vi "Convert Array to Image (Cam2) (SubVI).vi"(5 "Image Size":T2={"Height"=512, "Width"=512} {"Width" step=8; "Height" step=8}, 7 "Mode":enum16{"Camera", "Video"}(ring), 11 "Data In":T1) -> (0 "Compressed Image Size (%)":dbl, 3 "Image Out":T3)   [LabVIEW 2014]
uses:
  <vilib>/vision/Image Controls.llb/IMAQ Image.ctl
  Controls (HOST)/Image Size.ctl
  Controls (HOST)/Data to Disk Bundle.ctl
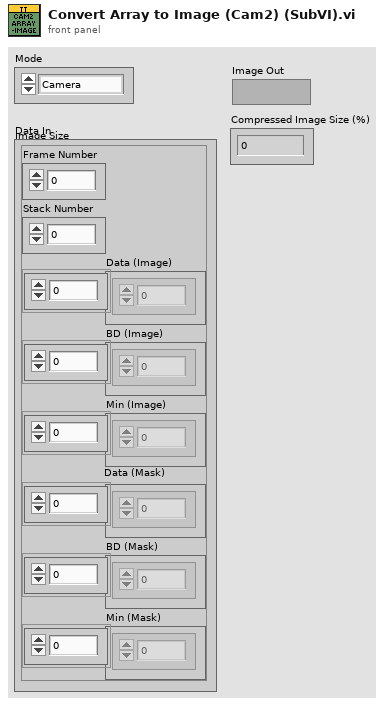
[diagram p1: front panel]
types:
  T1 = typedef "Data to Disk Bundle.ctl" = cluster{"Frame Number":u64, "Stack Number":u64, "Data (Image)":u64[], "BD (Image)":u8[], "Min (Image)":u8[], "Data (Mask)":u64[], "BD (Mask)":u8[], "Min (Mask)":u8[]}
  T2 = typedef "Image Size.ctl" = cluster{"Height":u16, "Width":u16}
  T3 = typedef "IMAQ Image.ctl" = refnum<image>
  T4 = enum16{"big-endian, network order", "native, host order", "little-endian"}
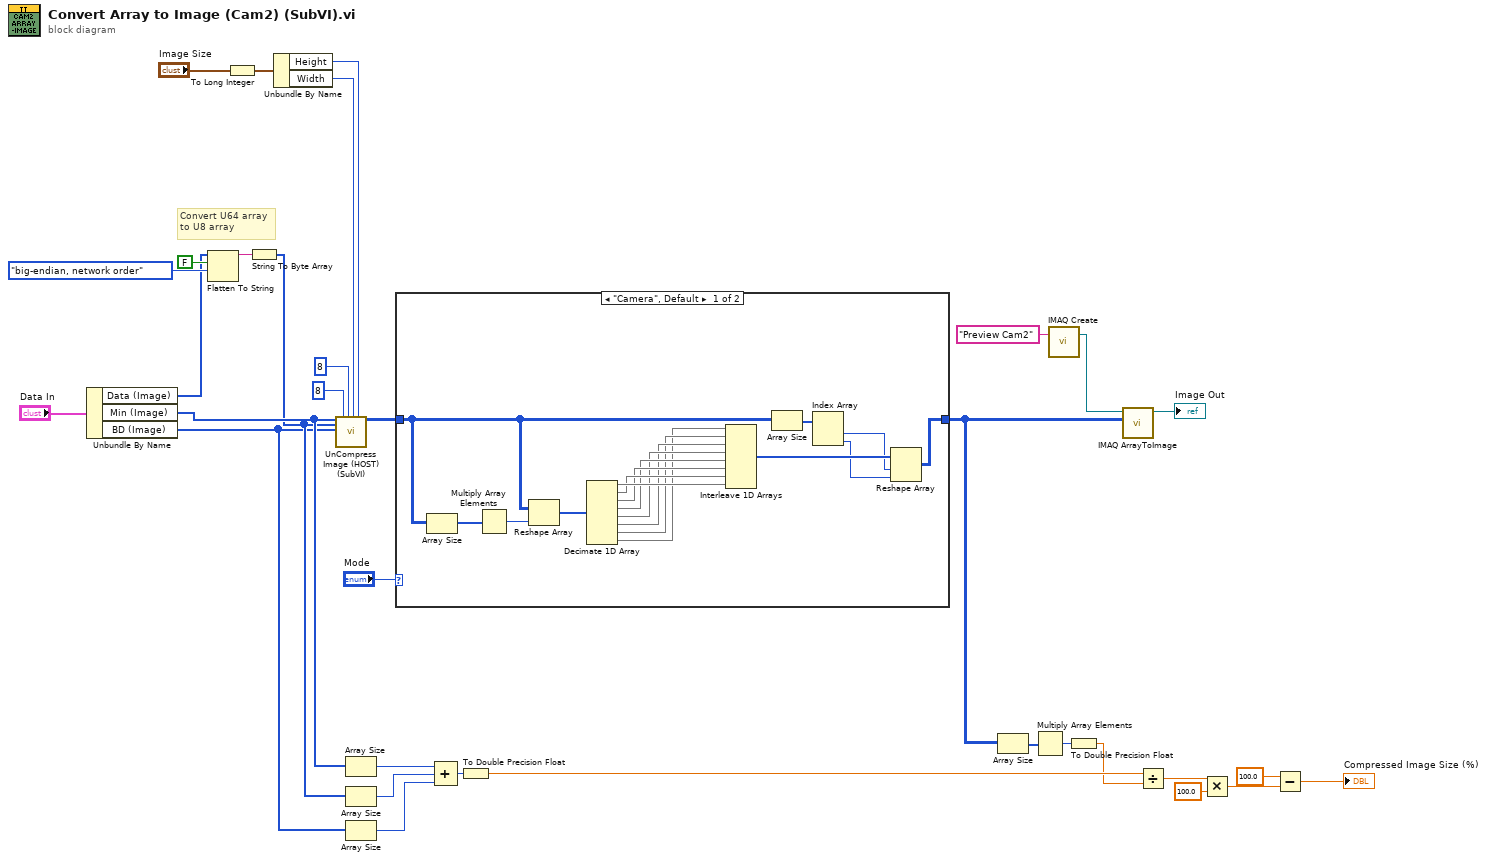
[diagram p0: block diagram]
diagram:
  # "Convert U64 array\nto U8 array"
  n1 = Unbundle By Name("Data In") -> ("Data (Image)"=w26:u64[], "Min (Image)"=w5:u8[], "BD (Image)"=w3:u8[])
  n2 = Flatten To String(anything=w26, prepend array or string size? (T)=FALSE, byte order (0:big-endian, network order)=T4."big-endian, network order") -> (data string=w28:string)  [unwired: 1 in, 2 out]
  n3 = To Long Integer(number="Image Size") -> (32bit integer=w22:cluster{"Height":i32, "Width":i32})
  n4 = String To Byte Array(string=w28) -> (unsigned byte array=w4:u8[])
  n5 = Unbundle By Name(w22) -> ("Height"=w21:i32, "Width"=w23:i32)
  n6 = call "UnCompress Image (HOST) (SubVI).vi"("Data Array"=w5, 1:w4, "Min. Array"=w3, "N Bits/Pixel"=u8 8, "Block Size"=8, "Image Width"=w23, "Image Height"=w21) -> ("Image Array Out"=w18:u8[][])  [unwired: 11 in, 1 out]
  n7 = Array Size(array=w5) -> (size(s)=w17:i32)
  n8 = Array Size(array=w4) -> (size(s)=w16:i32)
  n9 = Array Size(array=w3) -> (size(s)=w15:i32)
  n10 = case shown="\"Camera\", Default" "Mode" {
    tunnel: w18 -> [w38 w51]
    tunnel: [w34 w51] -> w6
    frame "Camera", Default {
      n11 = Array Size(array=w38) -> (size(s)=w50:i32[])
      n12 = Multiply Array Elements(1:w50) -> (0:w49:i32)
      n13 = Reshape Array(w38, w49) -> (w48:u8[])
      n14 = Decimate 1D Array(w48) -> (w47:u8[], w46:u8[], w45:u8[], w44:u8[], w43:u8[], w42:u8[], w41:u8[], w40:u8[])
      n15 = Interleave 1D Arrays(w40, w41, w42, w43, w44, w45, w46, w47) -> (w39:u8[])
      n16 = Array Size(array=w38) -> (size(s)=w37:i32[])
      n17 = Index Array(array=w37) -> (element #1=w36:i32, element #2=w35:i32)  [unwired: 2 in]
      n18 = Reshape Array(w39, w36, w35) -> (w34:u8[][])
    }
    frame "Video" {
    }
  }
  n19 = Compound Arithmetic op=ADD(w17, w16, w15) -> (w14:i32)
  n20 = To Double Precision Float(number=w14) -> (double precision float=w13:dbl)
  n21 = Array Size(array=w6) -> (size(s)=w12:i32[])
  n22 = Multiply Array Elements(1:w12) -> (0:w11:i32)
  n23 = call "IMAQ Create"("Image Name"="Preview Cam2") -> ("New Image"=w31:T3)  [unwired: 4 in, 1 out]
  n24 = To Double Precision Float(number=w11) -> (double precision float=w10:dbl)
  n25 = call "IMAQ ArrayToImage"("Image Pixels (U8)"=w6, "Image"=w31) -> ("Image Out"=→"Image Out":T3)  [unwired: 8 in, 1 out]
  n26 = Divide(x=w13, y=w10) -> (x/y=w9:dbl)
  n27 = Multiply(x=w9, y=100.0) -> (x*y=w7:dbl)
  n28 = Subtract(x=100.0, y=w7) -> (x-y=→"Compressed Image Size (%)":dbl)
